vi "Savitzky Golay Filter PtByPt with Derivative861.vi"(7 "initialize":bool, 9 "order polynomial":i32=1, 10 "side points":i32=15, 11 "x":dbl[](array[numeric]) format="%0.2f") -> (0 "error":i32, 2 "Filtered Derivative":dbl[](array[numeric]) format="%0.2f", 3 "Filtered x":dbl[](array[numeric]) format="%0.2f")   [LabVIEW 2014]
uses:
  <vilib>/Analysis/NI_AALBase.lvlib
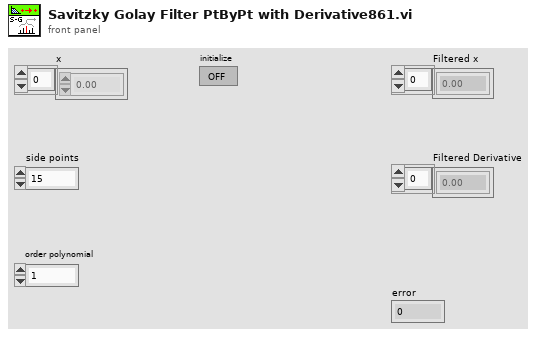
[diagram p1: front panel]
types:
  T1 = typedef "NI_Matrix.lvlib/RealMatrix.ctl" = dbl[][]
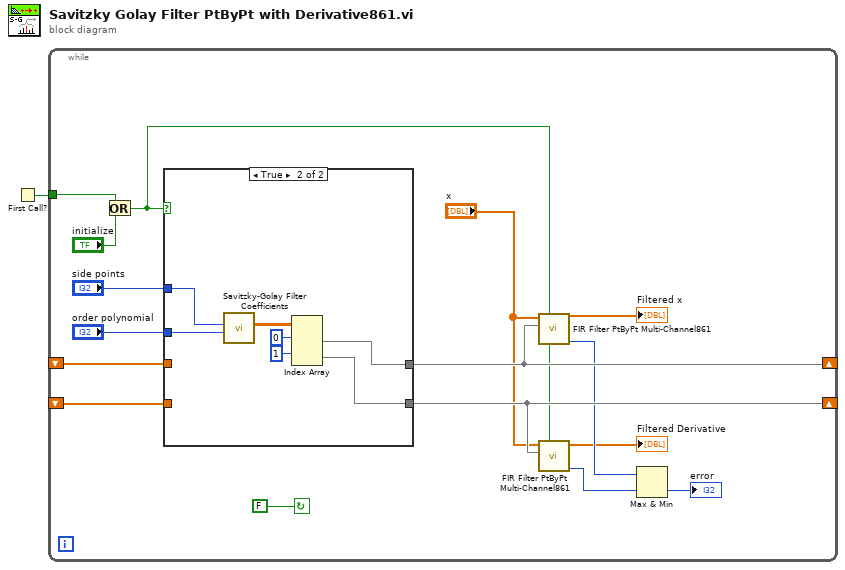
[diagram p0: block diagram]
diagram:
  n1 = First Call?() -> (First Call?: T/F=w1:bool)
  n2 = while {
    tunnel: w1 -> [w14]
    shift-left: _ -> [w17]
    shift-right: [w16] -> _
    shift-right: [w9] -> _
    shift-left: _ -> [w10]
    stop <- FALSE continue-if-true
    n3 = Or(x=w14, y="initialize") -> (x .or. y?=w5:bool)
    n4 = case shown="True" w5 {
      tunnel: [w19 w21] -> w16
      tunnel: w17 -> [w19 _]
      tunnel: "side points" -> [_ w25]
      tunnel: "order polynomial" -> [_ w26]
      tunnel: w10 -> [w18 _]
      tunnel: [w18 w20] -> w9
      frame False {
      }
      frame True {
        n5 = call <vilib>:"Savitzky-Golay Filter Coefficients.vi"("polynomial order"=w26, "side points"=w25) -> ("Differentiation Filters"=w24:T1)  [unwired: 2 in, 7 out]
        n6 = Index Array(array=w24, index (row) #1=0 ("index (row)"), index (row) #2=1 ("index (row)")) -> (element #1=w21:dbl[], element #2=w20:dbl[])  [unwired: 2 in]
      }
    }
    n7 = call "FIR Filter PtByPt Multi-Channel861.vi"("initialize"=w5, "Forward Coefficients"=w16, "x"="x") -> ("error"=w8:i32, "Filtered x"=→"Filtered x":dbl[])  [unwired: 1 in, 6 out]
    n8 = call "FIR Filter PtByPt Multi-Channel861.vi"("initialize"=w5, "Forward Coefficients"=w9, "x"="x") -> ("error"=w7:i32, "Filtered x"=→"Filtered Derivative":dbl[])  [unwired: 1 in, 6 out]
    n9 = Max & Min(x=w8, y=w7) -> (min(x,y)=→"error":i32)  [unwired: 1 out]
  }
